vi "Convert U32Cluster to U8 Representation.vi"(7 "Cluster Configuration":T1, 10 "U32 Cluster in":u32[](array[numeric])=[0, 0, 0]) -> (2 "U8 Cluster out":u8[](array[numeric]))   [LabVIEW 2018, in "FPGA Register IO.lvlib"]
uses:
  FPGA Register IO.lvlib
  TypeDefs/Cluster Configuration.ctl
  <userlib>/_OpenG.lib/lvdata/lvdata.llb/Type Descriptor__ogtk.ctl
  <vilib>/Utility/Data Type/Type Definitions/Data Type.ctl
  <vilib>/Utility/Data Type/NI_Data Type.lvlib
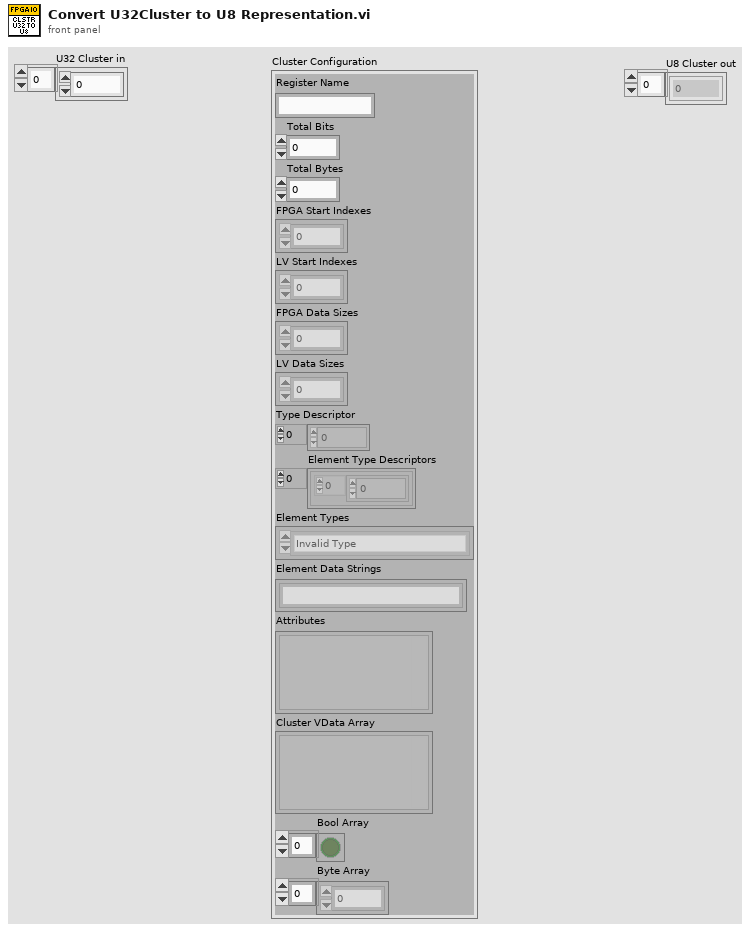
[diagram p1: front panel]
types:
  T1 = typedef "FPGA Register IO.lvlib/Cluster Configuration.ctl" = cluster{"Register Name":string, "Total Bits":i32, "Total Bytes":i32, "FPGA Start Indexes":i32[], "LV Start Indexes":i32[], "FPGA Data Sizes":i32[], "LV Data Sizes":i32[], "Type Descriptor":T2, "Element Type Descriptors":cluster{"Type Descriptor":T2}[], "Element Types":T3[], "Element Data Strings":string[], "Attributes":variant[], "Cluster VData Array":variant[], "Bool Array":bool[], "Byte Array":u8[]}
  T2 = typedef "Type Descriptor__ogtk.ctl" = i16[]
  T3 = typedef "NI_Data Type.lvlib/Data Type.ctl" = enum8{"Invalid Type", "Void", "I8", "I16", "I32", "I64", "U8", "U16", "U32", "U64", "Single Float", "Double Float", "Extended Float", "Single Complex", "Double Complex", "Extended Complex", "Enum U8", "Enum U16", "Enum U32", "Enum U64", "Single Float With Unit", "Double Float With Unit", "Extended Float With Unit", "Single Complex with Unit", "Double Complex with Unit", "Extended Complex with Unit", "Boolean", "String", "Path", "Picture", "Tag", "Array", "Cluster", "Variant", "LV Variant", "Waveform", "Timestamp", "Digital Waveform", "Digital Data", "ExpressData", "Refnum", "External Data", "VI", "Poly VI", "LabVIEW Class Instance", "Fixed Point"}
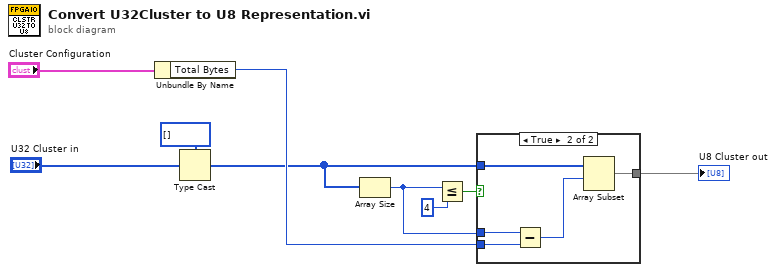
[diagram p0: block diagram]
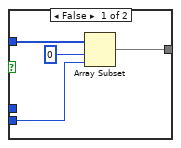
[diagram p2: hidden frame]
diagram:
  n1 = Unbundle By Name("Cluster Configuration") -> ("Total Bytes"=w8:i32)
  n2 = Type Cast(type=u8[] [] ("Cluster Byte Data"), x="U32 Cluster in") -> (*(type *) &x=w7:u8[])
  n3 = Array Size(array=w7) -> (size(s)=w4:i32)
  n4 = Less Or Equal?(x=w4, y=4) -> (x <= y?=w5:bool)
  n5 = case shown="True" w5 {
    tunnel: w8 -> [w12 w17]
    tunnel: w7 -> [w13 w16]
    tunnel: w4 -> [_ w15]
    tunnel: [w10 w14] -> w9
    frame False {
      n6 = Array Subset(array=w13, index=0, length=w12) -> (w10:u8[])
    }
    frame True {
      n7 = Subtract(x=w15, y=w17) -> (x-y=w18:i32)
      n8 = Array Subset(array=w16, index=w18) -> (w14:u8[])  [unwired: 1 in]
    }
  }
  "U8 Cluster out" <- w9
